vi "publishILCOutputs.vi"(8 "error in (no error)":errorcluster, 11 "Model in":refnum<class "Model.lvclass">) -> (0 "error out":errorcluster, 3 "Model out":refnum<class "Model.lvclass">)   [LabVIEW 2015, in "Model.lvclass"]
uses:
  Model.lvclass
  Model.lvclass/Model.ctl
  <userlib>/Common/ILC/ILC/ILC.lvclass/ILC.ctl
  UserEvents/UserEvents.lvclass/UserEvents.ctl
  UserEvents/UserEvents.lvclass
  <userlib>/Common/ILC/ILC/ILC.lvclass
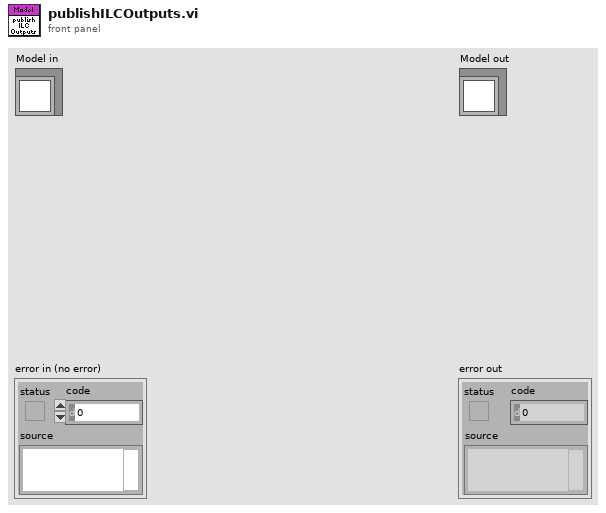
[diagram p1: front panel]
types:
  T1 = typedef "ILCCommon.lvlib/ILCTypedefs.lvlib/Outputs.ctl" = cluster{"Step & Direction":i16, "Blower RPM":u8, "PWM (SSR)":u8, "Ch1":u16, "Ch2":u16, "Ch3":u16, "Ch4":u16}
  T2 = typedef "FAMTTypedefs.lvlib/PubDataEvents.ctl" = cluster{"State":refnum<user-event>, "ErrorCode":refnum<user-event>, "ADC Outputs":refnum<user-event>, "InputData":refnum<user-event>, "ControllerData":refnum<user-event>, "TestStatus":refnum<user-event>, "LogPath":refnum<user-event>, "ILC Outputs":refnum<user-event>, "Scan Progress":refnum<user-event>}
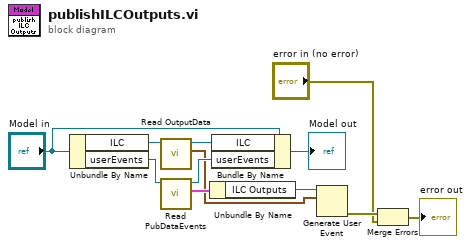
[diagram p0: block diagram]
diagram:
  n1 = Unbundle By Name("Model in") -> ("ILC"=w10:refnum<class "ILC.lvclass">, "userEvents"=w12:refnum<class "UserEvents.lvclass">)
  n2 = call <userlib>:"Read OutputData.vi"("ILC in"=w10) -> ("OutputData"=w1:T1, "ILC out"=w3:refnum<class "ILC.lvclass">)  [unwired: 9 in]
  n3 = call "Read PubDataEvents.vi"("UserEvents in"=w12) -> ("PubDataEvents"=w11:T2, "UserEvents out"=w2:refnum<class "UserEvents.lvclass">)  [unwired: 9 in]
  n4 = Unbundle By Name(w11) -> ("ILC Outputs"=w9:refnum<user-event>)
  n5 = Bundle By Name(cluster="Model in", "ILC"=w3, "userEvents"=w2) -> (→"Model out":refnum<class "Model.lvclass">)
  n6 = Generate User Event(user event=w9, event data cluster=w1) -> (error out=w8:errorcluster)  [unwired: 2 in, 1 out]
  n7 = Merge Errors(w8, "error in (no error)") -> (→"error out":errorcluster)
